vi "time us to s.vi"(10 "time (us)":fxp<+,48,48>) -> (2 "time (s)":dbl)   [LabVIEW 2017]
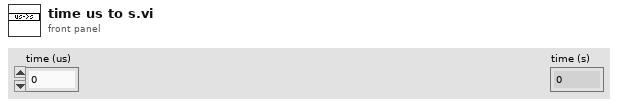
[diagram p1: front panel]
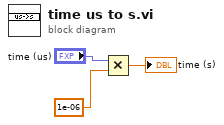
[diagram p0: block diagram]
diagram:
  n1 = Multiply(x="time (us)", y=1e-06) -> (x*y=→"time (s)":dbl)
